vi "Add.vi"(8 "error in":errorcluster, 10 "name":string="Ballard ARINC 429", 11 "target in":refnum<k24>) -> (0 "error out":errorcluster, 2 "Ballard ARINC 429 ref out":T1 format="%.0x", 3 "target out":refnum<k24>)   [LabVIEW 2020, in "Ballard ARINC 429 Scripting.lvlib"]
uses:
  Ballard ARINC 429 Scripting.lvlib
  NationalInstruments.VeriStand.SystemDefinitionAPI
  <vilib>/NI VeriStand/Custom Device API/Custom Device Item Ref.ctl
  Constants.vi
  <vilib>/NI VeriStand/Custom Device Tools/Custom Device Utility Library/Custom Device Utility Library.lvlib
  <vilib>/NI VeriStand/Custom Device API/Custom Device API.lvlib
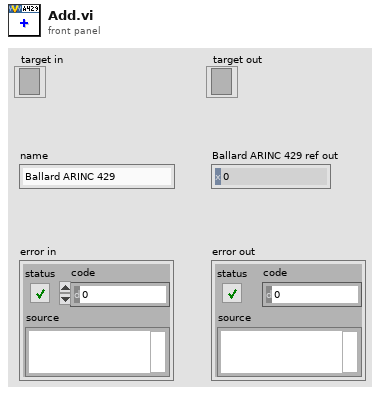
[diagram p1: front panel]
types:
  T1 = typedef "Custom Device API.lvlib/Custom Device Item Ref.ctl" = u64
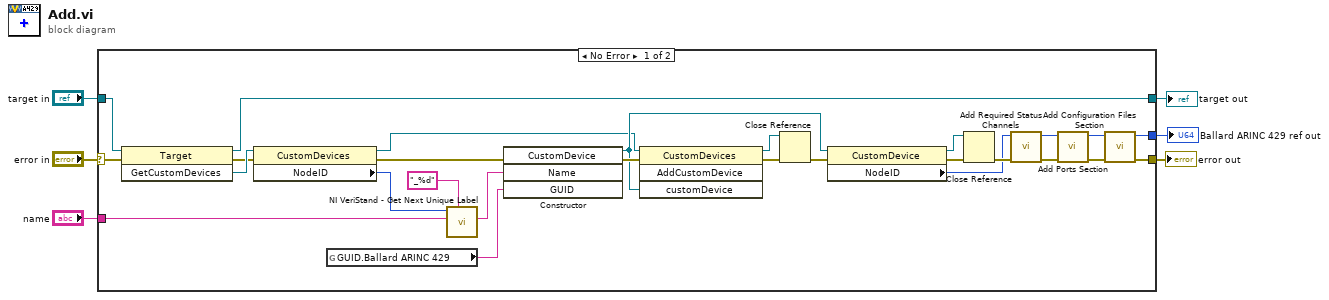
[diagram p0: block diagram]
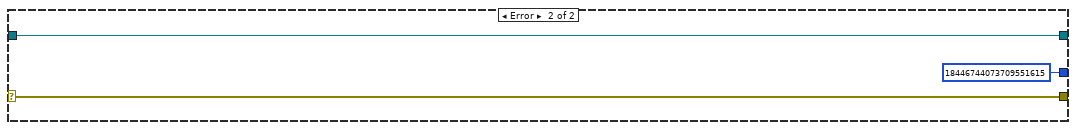
[diagram p2: hidden frame]
diagram:
  n1 = case shown="No Error" "error in" {
    selector: "error in" -> [w32 w36]
    tunnel: "target in" -> [w33 w35]
    tunnel: [w8 w36] -> w4
    tunnel: "name" -> [w20 _]
    tunnel: [w7 T1 18446744073709551615 ("Custom device Ref out")] -> w2
    tunnel: [w24 w35] -> w1
    frame No Error {
      n2 = invoke class="Target" method="GetCustomDevices"(reference=w33, error in=w32) -> (reference out=w24:refnum<k24>, error out=w17:errorcluster, "GetCustomDevices"=w22:refnum<k24>)  [unwired: 1 in]
      n3 = property class="CustomDevices"(reference=w22, error in=w17) -> (reference out=w15:refnum<k24>, error out=w16:errorcluster, "NodeID"=w21:u64)
      n4 = global read "Constants.vi" "GUID.Ballard ARINC 429"() -> (w23:string)
      n5 = call <vilib>:"NI VeriStand - Get Next Unique Label.vi"("format string"="_%d", "Label"=w20, "Parent Ref in"=w21) -> ("Label out"=w18:string)  [unwired: 5 in, 3 out]
      n6 = constructor class="CustomDevice"(error in=w16, "Name"=w18, "GUID"=w23) -> (reference out=w28:refnum<k24>, error out=w31:errorcluster)  [unwired: 2 in, 3 out]
      n7 = invoke class="CustomDevices" method="AddCustomDevice"(reference=w15, error in=w31, "customDevice"=w28) -> (reference out=w25:refnum<k24>, error out=w27:errorcluster)  [unwired: 1 in, 2 out]
      n8 = Close Reference(reference=w25, error in (no error)=w27) -> (error out=w26:errorcluster)
      n9 = property class="CustomDevice"(reference=w28, error in=w26) -> (reference out=w30:refnum<k24>, error out=w29:errorcluster, "NodeID"=w13:u64)
      n10 = Close Reference(reference=w30, error in (no error)=w29) -> (error out=w14:errorcluster)
      n11 = call "Add Required Status Channels.vi"("error in"=w14, "custom device ref"=w13) -> ("error out"=w11:errorcluster, "custom device ref out"=w12:T1)  [unwired: 7 in, 1 out]
      n12 = call "Add Ports Section.vi"("error in"=w11, "custom device ref"=w12) -> ("error out"=w9:errorcluster, "custom device ref out"=w10:T1)  [unwired: 7 in, 1 out]
      n13 = call "Add Configuration Files Section.vi"("error in"=w9, "Custom device Ref"=w10) -> ("error out"=w8:errorcluster, "Custom device Ref out"=w7:T1)  [unwired: 7 in, 1 out]
    }
    frame Error {
    }
  }
  "error out" <- w4
  "Ballard ARINC 429 ref out" <- w2
  "target out" <- w1
